vi "getParentVar.vi"(11 "Cow in":refnum<class "Cow.lvclass">) -> (2 "class name":string, 3 "Cow out":refnum<class "Cow.lvclass">)   [LabVIEW 2018]
uses:
  Cow.lvclass
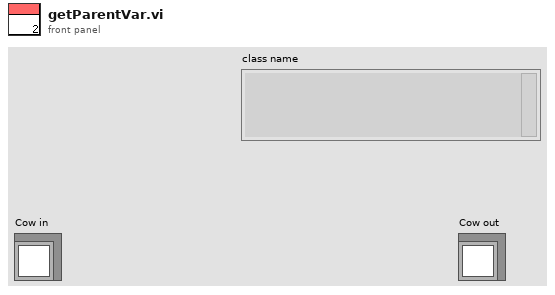
[diagram p1: front panel]
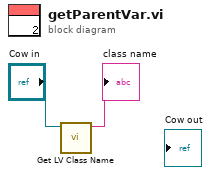
[diagram p0: block diagram]
diagram:
  n1 = call <vilib>:"Get LV Class Name.vi"("object"="Cow in") -> ("class name"=→"class name":string)  [unwired: 9 in, 1 out]
